vi "255 to 0.vi"(11 "255":string) -> (3 "0":string)   [LabVIEW 2013]
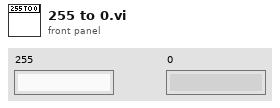
[diagram p1: front panel]
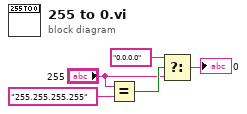
[diagram p0: block diagram]
diagram:
  n1 = Equal?(x="255", y="255.255.255.255") -> (x = y?=w4:bool)
  n2 = Select(t="0.0.0.0" ("y"), s=w4, f="255") -> (s? t:f=→"0":string)
